vi "Print to HTML MOD.vi"() -> ()   [LabVIEW 2017]
doc: "Saves the documentation for the VIs in an .llb to .html files. This example is similar to the Print LLB to HTML VI in this .llb, but you can use this example to select the components you want to print, such as the VI icon, connector pane, front panel, controls and indicators, VI hierarchy, and so on."
uses:
  <userlib>/_OpenG.lib/file/file.llb/Convert File Extension (String)__ogtk.vi
panel:
  out "HTML file":path
  # "Use the folder icons to browse to the desired file locations, set the Custom Details, then run the VI."
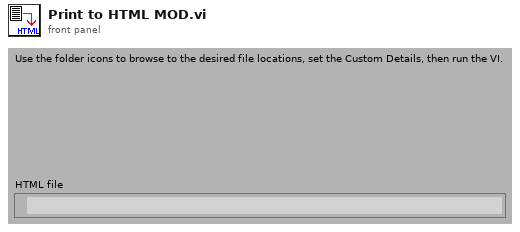
[diagram p1: front panel]
types:
  T1 = cluster{"Boolean 5":bool, "Boolean 6":bool, "Boolean 7":bool, "Boolean 8":bool, "Boolean 9":bool, "Boolean 2":bool, "Boolean":bool, "Boolean 3":bool, "Boolean 4":bool, "Boolean 10":bool, "Boolean 11":bool, "Boolean 12":bool, "Boolean 13":bool, "Boolean 14":bool, "Boolean 15":bool}
  T2 = enum32{"Custom", "Standard", "Using Panel", "Using SubVI", "Complete"}
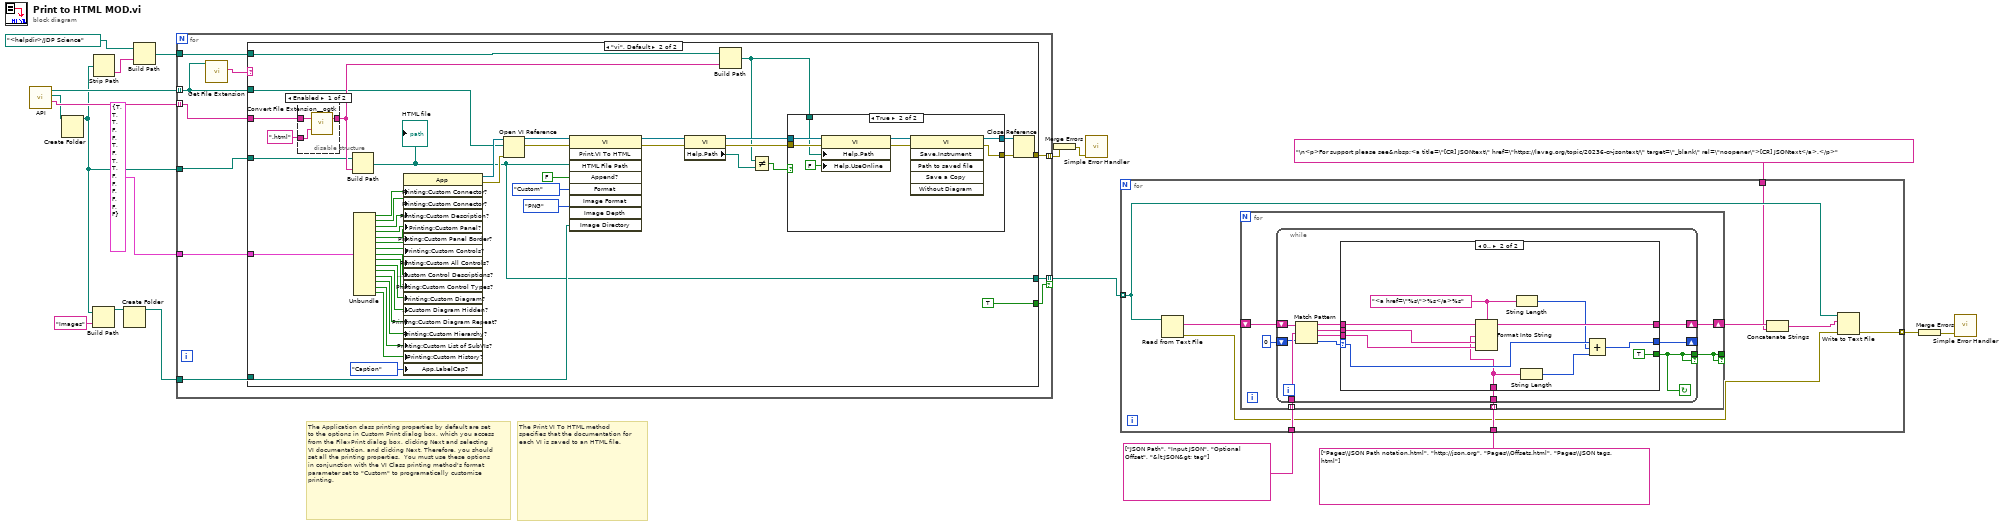
[diagram p0: block diagram]
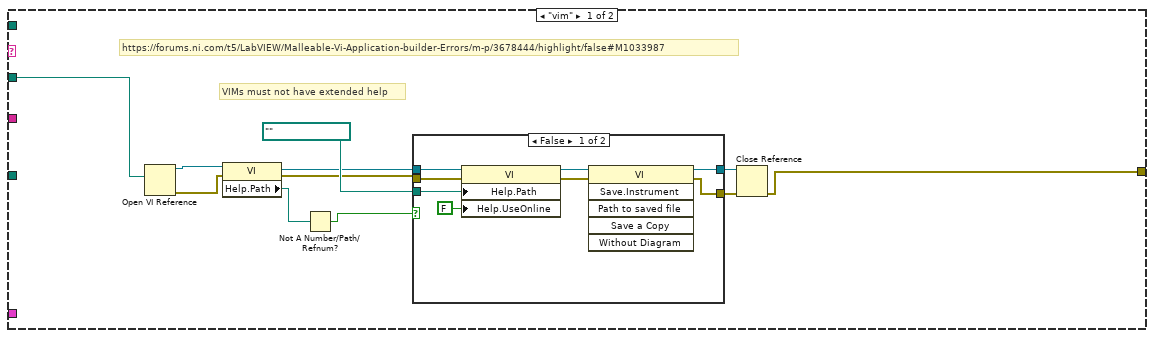
[diagram p2: hidden frame]
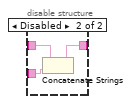
[diagram p5: hidden frame]
diagram:
  # "The Application class printing properties by default are set to the options in Custom Print dialog box, which you access from the File»Print dialog box, clicking Next and selecting VI documentation, and clicking Next. Therefore, you should set all the printing properties.  You must use these options in conjunction with the VI Class printing method's format parameter set to \"Custom\" to programatically customize printing."
  # "The Print VI To HTML method specifies that the documentation for each VI is saved to an HTML file."
  n1 = call "API.vi"() -> ("Names"=w15:string[], "Help Directory"=w12:path, "API"=w16:path[])  [unwired: 9 in]
  n2 = Create Folder(path (use dialog)=w12) -> (created path=w2:path)  [unwired: 2 in, 2 out]
  n3 = Build Path(base path=w2, name or relative path="Images") -> (appended path=w13:path)
  n4 = Strip Path(path=w2) -> (name=w10:string)  [unwired: 1 out]
  n5 = Create Folder(path (use dialog)=w13) -> (created path=w11:path)  [unwired: 2 in, 2 out]
  n6 = Build Path(base path=path "<helpdir>/JDP Science", name or relative path=w10) -> (appended path=w8:path)
  n7 = for {
    tunnel: w16 -> [w22] mode=indexing
    tunnel: w15 -> [w28] mode=indexing
    tunnel: [w29] -> w19 mode=indexing
    tunnel: w2 -> [w25]
    tunnel: T1 {"Boolean 5"=TRUE, "Boolean 6"=TRUE, "Boolean 7"=TRUE, "Boolean 8"=FALSE, "Boolean 9"=FALSE, "Boolean 2"=TRUE, "Boolean"=FALSE, "Boolean 3"=TRUE, "Boolean 4"=TRUE, "Boolean 10"=FALSE, "Boolean 11"=FALSE, "Boolean 12"=FALSE, "Boolean 13"=FALSE, "Boolean 14"=FALSE, "Boolean 15"=FALSE} ("Custom details") -> [w27]
    tunnel: w11 -> [w26]
    tunnel: w8 -> [w24]
    tunnel: [w23] -> w3 mode=indexing if=w20
    n8 = call <vilib>:"Get File Extension.vi"("file"=w22) -> ("lowercase file extension"=w21:string)  [unwired: 6 in, 4 out]
    n9 = case shown="\"vi\", Default" w21 {
      tunnel: [w32 w71] -> w29
      tunnel: w28 -> [_ w70]
      tunnel: w27 -> [_ w68]
      tunnel: w26 -> [_ w67]
      tunnel: w25 -> [_ w56]
      tunnel: w24 -> [_ w55]
      tunnel: [_ w53] -> w23
      tunnel: w22 -> [w38 w52]
      tunnel: [_ TRUE] -> w20
      frame "vim" {
        # "VIMs must not have extended help"
        # "https://forums.ni.com/t5/LabVIEW/Malleable-Vi-Application-builder-Errors/m-p/3678444/highlight/false#M1033987"
        n10 = Open VI Reference(vi path=w38) -> (vi reference=w35:refnum<vi>, error out=w33:errorcluster)  [unwired: 5 in]
        n11 = property class="VI"(reference=w35, error in=w33) -> (reference out=w36:refnum<vi>, error out=w34:errorcluster, "Help.Path"=w31:path)
        n12 = Not A Number/Path/Refnum?(number/path/refnum=w31) -> (NaN/Path/Refnum?=w30:bool)
        n13 = case shown="False" w30 {
          tunnel: w36 -> [w46 w50]
          tunnel: w34 -> [w42 w49]
          tunnel: [w45 w50] -> w40
          tunnel: [w43 w49] -> w39
          tunnel: path "" ("Help:Document Path") -> [w41 _]
          frame False {
            n14 = property class="VI"(reference=w46, error in=w42, "Help.Path"=w41, "Help.UseOnline"=FALSE ("Help:Use Web URL")) -> (reference out=w48:refnum<vi>, error out=w44:errorcluster)
            n15 = invoke class="VI" method="Save.Instrument"(reference=w48, error in=w44) -> (reference out=w45:refnum<vi>, error out=w43:errorcluster)  [unwired: 4 in, 4 out]
          }
          frame True {
          }
        }
        n16 = Close Reference ("Close LV Object Reference")(reference=w40, error in (no error)=w39) -> (error out=w32:errorcluster)
      }
      frame "vi", Default {
        n17 = disable-structure shown="Enabled" {
          disable-tunnel: w70 -> [w106 w108]
          disable-tunnel: ".html" ("replace string (\"\")") -> [w105 w109]
          disable-tunnel: [w104 w107] -> w66
          frame Enabled {
            n18 = call-poly <userlib>:"Convert File Extension__ogtk.vi"("new ending (none)"=w105, "file name"=w106) -> ("new filename"=w104:string)  [unwired: 1 out]
          }
          frame Disabled {
            n19 = Concatenate Strings(w108, w109) -> (w107:string)
          }
        }
        n20 = Build Path(base path=w56, name or relative path=w66) -> (appended path=w53:path)
        "HTML file" <- w53
        n21 = Unbundle "Unbundle"(w68) -> ("Boolean 5"=w87:bool, "Boolean 6"=w86:bool, "Boolean 7"=w85:bool, "Boolean 8"=w84:bool, "Boolean 9"=w83:bool, "Boolean 2"=w82:bool, "Boolean"=w81:bool, "Boolean 3"=w80:bool, "Boolean 4"=w79:bool, "Boolean 10"=w78:bool, "Boolean 11"=w77:bool, "Boolean 12"=w76:bool, "Boolean 13"=w75:bool, "Boolean 14"=w74:bool, "Boolean 15"=w73:bool)
        n22 = property on="Property Node" class="App"("Printing:Custom Connector?"=w87, "Printing:Custom Connector?"=w86, "Printing:Custom Description?"=w85, "Printing:Custom Panel?"=w84, "Printing:Custom Panel Border?"=w83, "Printing:Custom Controls?"=w82, "Printing:Custom All Controls?"=w81, "Printing:Custom Control Descriptions?"=w80, "Printing:Custom Control Types?"=w79, "Printing:Custom Diagram?"=w78, "Printing:Custom Diagram Hidden?"=w77, "Printing:Custom Diagram Repeat?"=w76, "Printing:Custom Hierarchy?"=w75, "Printing:Custom List of SubVIs?"=w74, "Printing:Custom History?"=w73, "App.LabelCap?"=enum16{"Label", "Caption", "Caption[Label]"}."Caption" ("Printing:Custom Control Label/Caption?")) -> (reference out=w89:refnum<vi>, error out=w88:errorcluster)  [unwired: 2 in]
        n23 = Open VI Reference(application reference (local)=w89, vi path=w52, error in (no error)=w88) -> (vi reference=w93:refnum<vi>, error out=w92:errorcluster)  [unwired: 3 in]
        n24 = invoke class="VI" method="Print.VI To HTML"(reference=w93, error in=w92, "HTML File Path"=w53, "Append?"=FALSE, "Format"=T2."Custom", "Image Format"=enum32{"PNG", "JPEG", "GIF"}."PNG", "Image Directory"=w67) -> (reference out=w64:refnum<vi>, error out=w65:errorcluster)  [unwired: 2 in, 7 out]
        n25 = property class="VI"(reference=w64, error in=w65) -> (reference out=w63:refnum<vi>, error out=w62:errorcluster, "Help.Path"=w60:path)
        n26 = Build Path(base path=w55, name or relative path=w66) -> (appended path=w61:path)
        n27 = Not Equal?(x=w61, y=w60) -> (x != y?=w57:bool)
        n28 = case shown="True" w57 {
          tunnel: w63 -> [w95 w101]
          tunnel: w62 -> [w94 w100]
          tunnel: w61 -> [_ w99]
          tunnel: [w95 w98] -> w59
          tunnel: [w94 w96] -> w58
          frame False {
          }
          frame True {
            n29 = property class="VI"(reference=w101, error in=w100, "Help.Path"=w99, "Help.UseOnline"=FALSE ("Help:Use Web URL")) -> (reference out=w103:refnum<vi>, error out=w97:errorcluster)
            n30 = invoke class="VI" method="Save.Instrument"(reference=w103, error in=w97) -> (reference out=w98:refnum<vi>, error out=w96:errorcluster)  [unwired: 4 in, 4 out]
          }
        }
        n31 = Close Reference ("Close LV Object Reference")(reference=w59, error in (no error)=w58) -> (error out=w71:errorcluster)
      }
    }
  }
  n32 = Merge Errors(w19) -> (w18:errorcluster)
  n33 = call <vilib>:"Simple Error Handler.vi"("error in (no error)"=w18) -> ()  [unwired: 4 in, 5 out]
  n34 = for {
    tunnel: w3 -> [w114] mode=indexing
    tunnel: string[] ["JSON Path", "Input JSON", "Optional Offset", "&lt;JSON&gt; tag"] ("regular expression") -> [w117]
    tunnel: string[] ["Pages\\JSON Path notation.html", "http://json.org", "Pages\\Offsets.html", "Pages\\JSON tags.html"] ("regular expression") -> [w116]
    tunnel: [w112] -> w4 mode=indexing
    tunnel: "\n<p>For support please see&nbsp;<a title=\"[CR] JSONtext\" href=\"https://lavag.org/topic/20236-cr-jsontext/\" target=\"_blank\" rel=\"noopener\">[CR] JSONtext</a>.</p>" ("string") -> [w110]
    n35 = Read from Text File(file (use dialog)=w114) -> (text=w118:string, error out=w113:errorcluster)  [unwired: 3 in, 2 out]
    n36 = for {
      tunnel: w117 -> [w123] mode=indexing
      shift-right: [w122] -> w115
      shift-left: w118 -> [w124]
      tunnel: w116 -> [w121] mode=indexing
      tunnel: [w120] -> _ if=w120
      n37 = while {
        tunnel: w123 -> [w134]
        tunnel: w121 -> [w128]
        tunnel: [w125] -> w120 if=w125
        shift-right: [w132] -> w122
        shift-left: w124 -> [w135]
        shift-right: [w127] -> _
        shift-left: 0 ("offset past match") -> [w126]
        stop <- w125 continue-if-true
        n38 = Match Pattern(string=w135, regular expression=w134, offset (0)=w126) -> (before substring=w131:string, match substring=w129:string, after substring=w130:string, offset past match=w133:i32)
        n39 = case shown="0.." w133 {
          selector: w133 -> [_ w142]
          tunnel: [w136 w144] -> w132
          tunnel: w131 -> [w136 w147]
          tunnel: w130 -> [_ w145]
          tunnel: w129 -> [_ w146]
          tunnel: w128 -> [_ w140]
          tunnel: [_ TRUE] -> w125
          tunnel: [_ w141] -> w127
          frame Default {
          }
          frame 0.. {
            w138 = "<a href=\"%s\">%s</a>%s" ("format string")
            n40 = Format Into String(format string=w138, initial string=w147, w140, w146, w145) -> (resulting string=w144:string)  [unwired: 1 in, 1 out]
            n41 = String Length(string=w138) -> (length=w137:i32)
            n42 = String Length(string=w140) -> (length=w139:i32)
            n43 = Compound Arithmetic op=ADD(w142, w137, w139) -> (w141:i32)
          }
        }
      }
    }
    n44 = Concatenate Strings(w115, w110) -> (w111:string)
    n45 = Write to Text File(file (use dialog)=w114, text=w111, error in=w113) -> (error out=w112:errorcluster)  [unwired: 1 in, 2 out]
  }
  n46 = Merge Errors(w4) -> (w5:errorcluster)
  n47 = call <vilib>:"Simple Error Handler.vi"("error in (no error)"=w5) -> ()  [unwired: 4 in, 5 out]
